vi "Run.vi"(7 "Team Index":i32, 8 "Column":i32, 9 "Row":i32, 10 "View":i32[](array[numeric]) caption="View (Team Index, -1: empty)", 11 "Test In":refnum<class "Pattern 4.lvclass">) -> (0 "Replicated":refnum<class "Square.lvclass">, 1 "Direction":T1, 2 "Action":T2, 3 "Test Out":refnum<class "Square.lvclass">)   [LabVIEW 2020, in "Pattern 4.lvclass"]
uses:
  Pattern 4.lvclass
  Pattern 4.lvclass/Pattern 4.ctl
  Type Defs/Action Enum.ctl
  Type Defs/SB Type Defs.lvlib
  Squares/Common/Common.lvlib
  C:/dev/IlluminatedG/sol-squarebattle/Square/Square.lvclass
  C:/dev/IlluminatedG/sol-squarebattle/Documents/Patterns/Pattern 4/Pattern 4.lvclass
  Square/Square.lvclass
  Type Defs/Direction Enum.ctl
panel:
  # "NW\nN\nNE\nE\nSE\nS\nSW\nW"
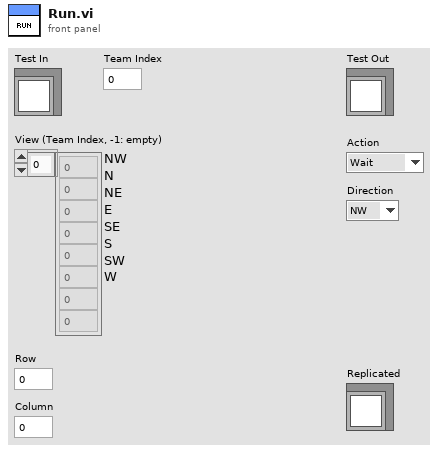
[diagram p1: front panel]
types:
  T1 = typedef "SB Type Defs.lvlib/Direction Enum.ctl" = enum16{"NW", "N", "NE", "E", "SE", "S", "SW", "W"}
  T2 = typedef "SB Type Defs.lvlib/Action Enum.ctl" = enum16{"Wait", "Move", "Attack", "Replicate"}
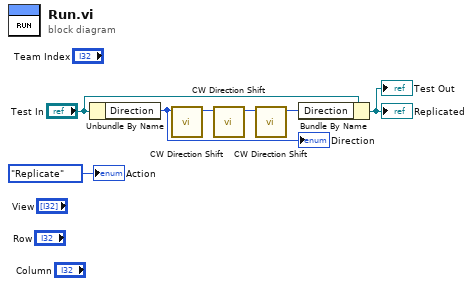
[diagram p0: block diagram]
diagram:
  n1 = Unbundle By Name("Test In") -> ("Direction"=w1:T1)
  "Direction" <- w1
  n2 = call "CW Direction Shift.vi"("Direction"=w1) -> ("Numeric"=w3:i32)  [unwired: 10 in]
  n3 = call "CW Direction Shift.vi"("Direction"=w3) -> ("Numeric"=w2:i32)  [unwired: 10 in]
  n4 = call "CW Direction Shift.vi"("Direction"=w2) -> ("Numeric"=w4:i32)  [unwired: 10 in]
  n5 = Bundle By Name(cluster="Test In", "Direction"=w4) -> (→"Test Out" →"Replicated":refnum<class "Pattern 4.lvclass">)
  "Action" <- Action_Enum."Replicate" ("Action")
